vi "Read Port Register.vi"(11 "DIO in":refnum<class "Digital IO.lvclass">) -> (3 "port register":u8)   [LabVIEW 2017, in "Digital IO.lvlib" / "Digital IO.lvclass"]
uses:
  Digital IO.lvclass
  Digital IO.lvclass/Digital IO.ctl
  <vilib>/rvi/DataTransferAndStorage/Container/Common/niFpgaContainerExecOnDevCompGetState.vi
  <vilib>/rvi/Emulation/niFpgaEmulationIsFPGAContextNoSignature.vi
  <vilib>/rvi/DataTransferAndStorage/Container/Common/niFpgaContainerGetUniqueNameForEmu.vi
  <vilib>/rvi/eio/common/nirviEmuReportErrorAndStop.vi
  <vilib>/rvi/Emulation/niFpgaSctlEmulationGetInTimedLoop.vi
  <vilib>/rvi/Emulation/niFpgaProcessEmulError.vi
  <vilib>/rvi/DataTransferAndStorage/Container/XNode/niFpgaContainer.xnode
  <vilib>/rvi/DataTransferAndStorage/Handshake/Emulation/niFpgaHandshakeEmulationRefIn.vi
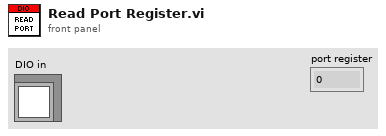
[diagram p1: front panel]
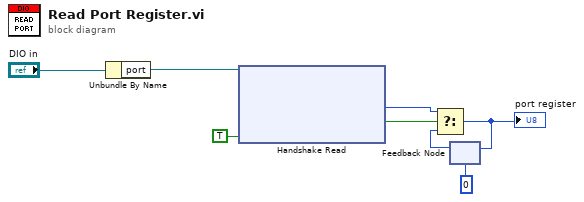
[diagram p0: block diagram]
diagram:
  n1 = Unbundle By Name("DIO in") -> ("port"=w7:refnum<k21>)
  n2 = xnode ("Handshake Read")("Ready for Output"=TRUE, "Handshake In"=w7) -> ("Data"=w5:u8, "Output Valid"=w6:bool)  [unwired: 1 out]
  n3 = feedback #1(u8 0 ("Data")) -> (w4:u8)
  n4 = Select(t=w5, s=w6, f=w4) -> (s? t:f=w3:u8)
  "port register" <- w3
  n5 = feedback-in #1(w3) -> ()
